vi "Move_PicoMotors.vi"(5 "PicoMotor":u16(ring) items=["Z (AO7)"], 11 "APPROXIMATE Distance (µm)":dbl min=0.0) -> ()   [LabVIEW 2023]
uses:
  Sub_Vi/TypeDefs/Settings.ctl
  Sub_Vi/TypeDefs/WayPointCluster.ctl
  Sub_Vi/TypeDefs/ChangeOnFly.ctl
  Settings.vi
panel:
  in  "Start scan Button":bool
  in  "stop 2":bool
  in  "ChangeonFly":T1
  in  "Direction\n (on = positive/up, off = negative/down)":bool=TRUE
  in  "WayPointCluster":T2
  in  "SettingsCluster":T3={"Sample Rate (us)"=1, "Samples Per Data Point (int, power of 2)"=1000, "DistanceToBulk (um)"=-1.0, "HoldTimeScaler"=40000, "SaveData"=TRUE, "DistanceToBulk (um) 2"=-1.0, "DistanceToBulk (um) 3"=-1.0}
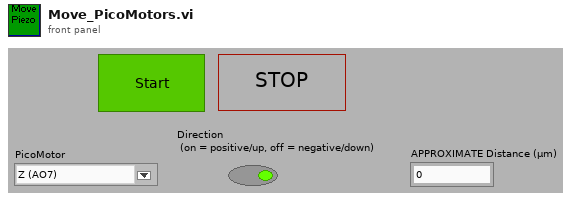
[diagram p1: front panel]
types:
  T1 = typedef "ChangeOnFly.ctl" = cluster{"Stop (boolean)":refnum<vi>, "Pause (boolean)":refnum<vi>, "EndCurrentLine (boolean)":refnum<vi>, "max movement per update step (Interger, nm)":refnum<vi>, "P (float, arb)":refnum<vi>, "Feedback set point (double, Amps)":refnum<vi>, "Voltage (double, V)":refnum<vi>, "Feedback set point 2 (double, Amps)":refnum<vi>, "Stop on Greater Than 2? (boolean)":refnum<vi>, "Stop on Greater Than? (boolean)":refnum<vi>, "Voltage 2 (double, V)":refnum<vi>, "Feedback Type (enum)":refnum<vi>, "Feedback Type 2 (enum)":refnum<vi>}
  T2 = typedef "WayPointCluster.ctl" = cluster{"X (um)":dbl[], "Y (um)":dbl[], "Z (um)":dbl[], "V (V)":dbl[], "X Velocity (um s-1)":dbl[], "Y Velocity (um s-1)":dbl[], "Z Velocity (um s-1)":dbl[], "V Velocity (V s-1)":dbl[], "FeedBack Type (enum)":u16[], "Move X (boolean)":bool[], "Move Y (boolean)":bool[], "Move Z (boolean)":bool[], "Move V (boolean)":bool[], "Jump V (boolean)":bool[], "Hold (boolean)":bool[], "Hold Time":u32[], "V2 (V)":dbl[], "Move V2":bool[], "V2 Velocity (V s-1)":dbl[], "Jump V2 (boolean)":bool[], "Update z Position delta (ms)":i16[], "Hold Feedback1":bool[], "Move Z PicoMotor":bool[], " Z PicoMotor Direction":bool[], "DIO0":bool[]}
  T3 = typedef "Settings.ctl" = cluster{"Sample Rate (us)":u32, "Samples Per Data Point (int, power of 2)":i16, "DistanceToBulk (um)":dbl, "HoldTimeScaler":u64, "SaveData":bool, "DistanceToBulk (um) 2":dbl, "DistanceToBulk (um) 3":dbl}
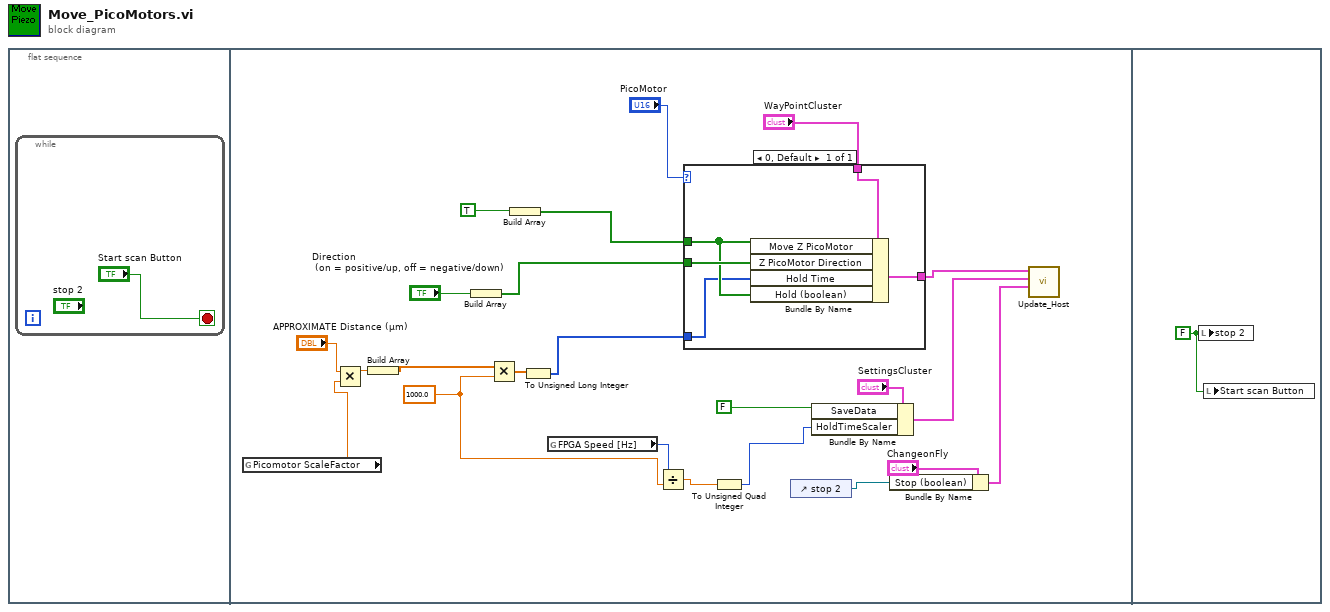
[diagram p0: block diagram]
diagram:
  n1 = flat-sequence {
    frame #0 {
      n2 = while {
        stop <- "Start scan Button" stop-if-true
      }
    }
    frame #1 {
      w4 = 1000.0
      n3 = global read "Settings.vi" "Picomotor ScaleFactor"() -> (w2:dbl)
      n4 = Multiply(x="APPROXIMATE Distance (µm)", y=w2) -> (x*y=w7:dbl)
      n5 = Build Array(w7) -> (w17:dbl[])
      n6 = Build Array("Direction\n (on = positive/up, off = negative/down)") -> (w12:bool[])
      n7 = Multiply(x=w17, y=w4) -> (x*y=w18:dbl[])
      n8 = Build Array(TRUE ("Set X")) -> (w14:bool[])
      n9 = To Unsigned Long Integer(number=w18) -> (unsigned 32bit integer=w16:u32[])
      n10 = global read "Settings.vi" "FPGA Speed [Hz]"() -> (w5:i64)
      n11 = Divide(x=w5, y=w4) -> (x/y=w6:dbl)
      n12 = case shown="0, Default" "PicoMotor" {
        tunnel: "WayPointCluster" -> [w29]
        tunnel: [w28] -> w23
        tunnel: w16 -> [w25]
        tunnel: w14 -> [w26]
        tunnel: w12 -> [w27]
        frame 0, Default {
          n13 = Bundle By Name(cluster=w29, "Move Z PicoMotor"=w26, "Z PicoMotor Direction"=w27, "Hold Time"=w25, "Hold (boolean)"=w26) -> (w28:T2)
        }
      }
      n14 = To Unsigned Quad Integer(1:w6) -> (0:w3:u64)
      n15 = control-ref of="stop 2"() -> (w9:refnum<vi>)
      n16 = Bundle By Name(cluster="SettingsCluster", "SaveData"=FALSE ("Set X"), "HoldTimeScaler"=w3) -> (w19:T3)
      n17 = Bundle By Name(cluster="ChangeonFly", "Stop (boolean)"=w9) -> (w8:T1)
      n18 = call "Update_Host.vi"("ChangeonFly"=w8, "SettingsCluster"=w19, "WayPointCluster"=w23) -> ()  [unwired: 7 in]
    }
    frame #2 {
      w30 = FALSE ("stop 2")
      n19 = local write "stop 2"(w30) -> ()
      n20 = local write "Start scan Button"(w30) -> ()
    }
  }
